vi "GlobalGetKoherasLaserOnOff.vi"() -> ()   [LabVIEW 2013]
panel:
  out "GetKoherasLaser":bool
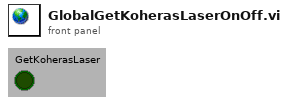
[diagram p1: front panel]
diagram:
